vi "Angle measurement.vi"(0 "Image":T6, 5 "Anglr Input Cluster":T5={"Meas ROI-1 After Transformation"={"Global Rectangle"=[], "Contours"=[]}, "Meas ROI-1 Scan/Search Direction"=2, "Meas ROI-1 Edge Options"={"Edge Polarity"=2, "Kernel Size"=5, "Width"=3, "Minimum Edge Strength"=50.0, "Interpolation Type"=enum."Zero Order", "Data Processing Method"=enum."Average"}, "Meas ROI-1 Line Options"={"Number of Lines"=1, "Type"=enum."First Edge Rake", "Min. Score"=0.0, "Max. Score"=1024.0, "Orientation"=0.0, "Angle Range"=20.0, "Angle Tolerance"=1.0, "Step Size"=10, "Min. SNR (db)"=3.0, "Min. Points (%)"=25.0, "Hough Iterations"=5}, "Refrence_ROI_After Tramsformation"={"Global Rectangle"=[], "Contours"=[]}, "Ref line Search Direction"=1, "Ref Line Options"={"Number of Lines"=1, "Type"=enum."First Edge Rake", "Min. Score"=0.0, "Max. Score"=1024.0, "Orientation"=0.0, "Angle Range"=20.0, "Angle Tolerance"=1.0, "Step Size"=10, "Min. SNR (db)"=3.0, "Min. Points (%)"=25.0, "Hough Iterations"=5}, "Ref Line Edge Options"={"Edge Polarity"=2, "Kernel Size"=5, "Width"=3, "Minimum Edge Strength"=50.0, "Interpolation Type"=enum."Zero Order", "Data Processing Method"=enum."Average"}} {"Ref Line Edge Options"."Edge Polarity" items=["All Edges", "Rising Edges", "Falling Edges"]; "Ref Line Edge Options"."Minimum Edge Strength" format="%.2f"; "Ref Line Edge Options"."Width" step=2; "Ref Line Edge Options"."Kernel Size" step=2; "Ref Line Options"."Min. Points (%)" min=0.0 max=100.0; "Ref Line Options"."Min. SNR (db)" min=0.0; "Ref Line Options"."Max. Score" min=0.0 max=1024.0; "Ref Line Options"."Min. Score" min=0.0 max=1024.0 step=1.0; "Ref line Search Direction" items=["Left to Right", "Right to Left", "Top to Bottom", "Bottom to Top"]; "Meas ROI-1 Line Options"."Min. Points (%)" min=0.0 max=100.0; "Meas ROI-1 Line Options"."Min. SNR (db)" min=0.0; "Meas ROI-1 Line Options"."Max. Score" min=0.0 max=1024.0; "Meas ROI-1 Line Options"."Min. Score" min=0.0 max=1024.0 step=1.0; "Meas ROI-1 Edge Options"."Edge Polarity" items=["All Edges", "Rising Edges", "Falling Edges"]; "Meas ROI-1 Edge Options"."Minimum Edge Strength" format="%.2f"; "Meas ROI-1 Edge Options"."Width" step=2; "Meas ROI-1 Edge Options"."Kernel Size" step=2; "Meas ROI-1 Scan/Search Direction" items=["Left to Right", "Right to Left", "Top to Bottom", "Bottom to Top"]}, 11 "error in":errorcluster) -> (4 "Angle":sgl, 6 "Image Out":T6, 15 "error out":errorcluster)   [LabVIEW 2019, in "Algorithm.lvclass"]
uses:
  FrameworkOverrides/Algorithm.lvclass
  <vilib>/vision/NI_Vision_Development_Module.lvlib
  <vilib>/vision/Image Controls.llb/IMAQ Image.ctl
  <vilib>/vision/Measure.llb/Edge Polarity.ctl
  <vilib>/vision/Measure.llb/Edge Options.ctl
  <vilib>/vision/Measure.llb/Straight Edge Process.ctl
  <vilib>/vision/Measure.llb/Straight Edge Options.ctl
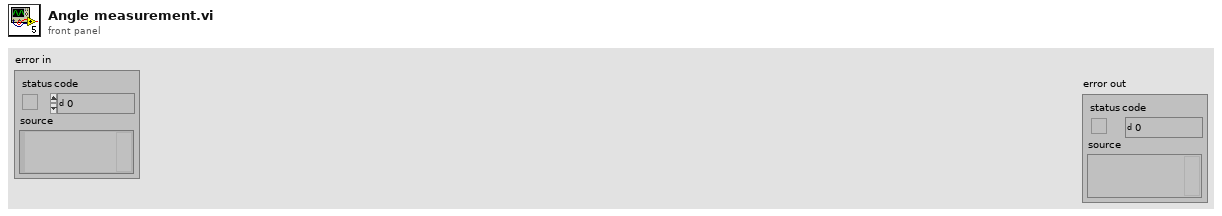
[diagram p1: front panel]
types:
  T1 = typedef "Edge Options.ctl" = cluster{"Edge Polarity":T2, "Kernel Size":u32, "Width":u32, "Minimum Edge Strength":sgl, "Interpolation Type":enum32{"Zero Order", "Bilinear", "Quadratic", "Cubic", "Bilinear Fixed"}, "Data Processing Method":enum32{"Average", "Median"}}
  T2 = typedef "Edge Polarity.ctl" = u32
  T3 = typedef "Straight Edge Options.ctl" = cluster{"Number of Lines":i32, "Type":T4, "Min. Score":dbl, "Max. Score":dbl, "Orientation":dbl, "Angle Range":dbl, "Angle Tolerance":dbl, "Step Size":u32, "Min. SNR (db)":dbl, "Min. Points (%)":dbl, "Hough Iterations":i32}
  T4 = typedef "Straight Edge Process.ctl" = enum32{"First Edge Rake", "Best Edge Rake", "Hough Edge Rake", "First Edge Projection", "Best Edge Projection"}
  T5 = cluster{"Meas ROI-1 After Transformation":cluster{"Global Rectangle":i32[], "Contours":cluster{"ID":enum32{"External", "Internal"}, "Type":u32, "Coordinates":i32[]}[]}, "Meas ROI-1 Scan/Search Direction":u32, "Meas ROI-1 Edge Options":T1, "Meas ROI-1 Line Options":T3, "Refrence_ROI_After Tramsformation":cluster{"Global Rectangle":i32[], "Contours":cluster{"ID":enum32{"External", "Internal"}, "Type":u32, "Coordinates":i32[]}[]}, "Ref line Search Direction":u32, "Ref Line Options":T3, "Ref Line Edge Options":T1}
  T6 = typedef "IMAQ Image.ctl" = refnum<image>
  T7 = cluster{"Global Rectangle":i32[], "Contours":cluster{"ID":enum32{"External", "Internal"}, "Type":u32, "Coordinates":i32[]}[]}
  T8 = cluster{"Point1 (Pixels)":cluster{"X":sgl, "Y":sgl}, "Point2 (Pixels)":cluster{"X":sgl, "Y":sgl}, "Point1 (Real-World)":cluster{"X":sgl, "Y":sgl}, "Point2 (Real-World)":cluster{"X":sgl, "Y":sgl}, "Angle (Pixel)":dbl, "Angle (Real-World)":dbl, "Score":dbl, "Straightness":dbl, "Average SNR (db)":dbl, "Calibration Valid":bool}[]
  T9 = cluster{"Point1 (Pixels)":cluster{"X":sgl, "Y":sgl}, "Point2 (Pixels)":cluster{"X":sgl, "Y":sgl}, "Point1 (Real-World)":cluster{"X":sgl, "Y":sgl}, "Point2 (Real-World)":cluster{"X":sgl, "Y":sgl}, "Angle (Pixel)":dbl, "Angle (Real-World)":dbl, "Score":dbl, "Straightness":dbl, "Average SNR (db)":dbl, "Calibration Valid":bool}
  T10 = cluster{"Point1 (Pixels)":cluster{"X":sgl, "Y":sgl}, "Point2 (Pixels)":cluster{"X":sgl, "Y":sgl}, "Point1 (Pixels)":cluster{"X":sgl, "Y":sgl}, "Point2 (Pixels)":cluster{"X":sgl, "Y":sgl}}
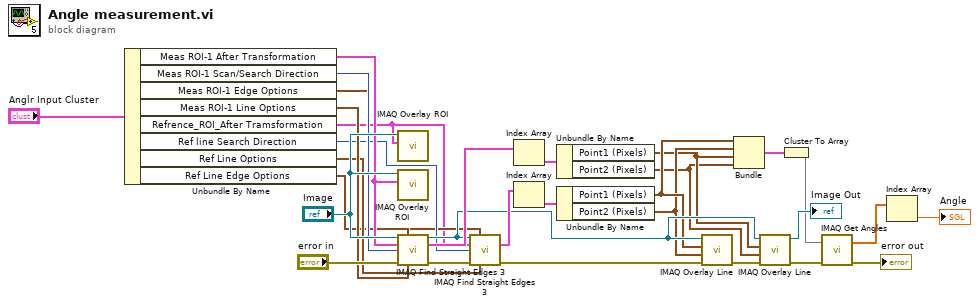
[diagram p0: block diagram]
diagram:
  n1 = Unbundle By Name("Anglr Input Cluster") -> ("Meas ROI-1 After Transformation"=w15:T7, "Meas ROI-1 Scan/Search Direction"=w14:u32, "Meas ROI-1 Edge Options"=w13:T1, "Meas ROI-1 Line Options"=w12:T3, "Refrence_ROI_After Tramsformation"=w8:T7, "Ref line Search Direction"=w11:u32, "Ref Line Options"=w10:T3, "Ref Line Edge Options"=w9:T1)
  n2 = call "IMAQ Overlay ROI"("ROI Descriptor"=w8, "Image"="Image") -> ()  [unwired: 8 in, 2 out]
  n3 = call "IMAQ Overlay ROI"("ROI Descriptor"=w15, "Image"="Image") -> ()  [unwired: 8 in, 2 out]
  n4 = call "IMAQ Find Straight Edges 3"("Image"="Image", "Edge Options"=w13, "ROI Descriptor"=w15, "Search Direction"=w14, "error in (no error)"="error in", "Line Options"=w12) -> ("Image (duplicate)"=w18:T6, "Straight Edges"=w26:T8, "error out"=w28:errorcluster)  [unwired: 5 in, 2 out]
  n5 = call "IMAQ Find Straight Edges 3"("Image"=w18, "Edge Options"=w9, "ROI Descriptor"=w8, "Search Direction"=w11, "error in (no error)"=w28, "Line Options"=w10) -> ("Straight Edges"=w24:T8, "error out"=w21:errorcluster)  [unwired: 5 in, 3 out]
  n6 = Index Array(array=w26) -> (element=w27:T9)  [unwired: 1 in]
  n7 = Index Array(array=w24) -> (element=w25:T9)  [unwired: 1 in]
  n8 = Unbundle By Name(w27) -> ("Point1 (Pixels)"=w4:cluster{"X":sgl, "Y":sgl}, "Point2 (Pixels)"=w3:cluster{"X":sgl, "Y":sgl})
  n9 = Unbundle By Name(w25) -> ("Point1 (Pixels)"=w6:cluster{"X":sgl, "Y":sgl}, "Point2 (Pixels)"=w5:cluster{"X":sgl, "Y":sgl})
  n10 = call "IMAQ Overlay Line"("error in (no error)"=w21, "End Point"=w5, "Start Point"=w6, "Image"=w18) -> ("error out"=w20:errorcluster)  [unwired: 6 in, 1 out]
  n11 = Bundle("Point1 (Pixels)"=w6, "Point2 (Pixels)"=w5, "Point1 (Pixels)"=w4, "Point2 (Pixels)"=w3) -> (w2:T10)  [unwired: 1 in]
  n12 = call "IMAQ Overlay Line"("error in (no error)"=w20, "End Point"=w3, "Start Point"=w4, "Image"=w18) -> ("error out"=w7:errorcluster, "Image Out"=→"Image Out":T6)  [unwired: 6 in]
  n13 = Cluster To Array(cluster=w2) -> (array=w1:cluster{"X":sgl, "Y":sgl}[])
  n14 = call "IMAQ Get Angles"("error in (no error)"=w7, "Points"=w1) -> ("error out"=→"error out":errorcluster, "Angles (deg)"=w23:sgl[])  [unwired: 3 in, 1 out]
  n15 = Index Array(array=w23) -> (element=→"Angle":sgl)  [unwired: 1 in]
